vi "GetNodeHeirarchyArray_recursively.vi"(8 "error in (no error)":errorcluster, 9 "2D Array_All Paths":refnum<vi>, 10 "Nodes heirarchy IN (Leave EMPTY - used for recursion)":string[](array[string]), 11 "Node IN":refnum<k20>) -> (0 "error out":errorcluster)   [LabVIEW 2012]
doc: "SciScan 1.2 160622"
uses:
  <resource>/objmgr/DOMUserDefRef.rc
  <vilib>/xml/NI_XML.lvlib
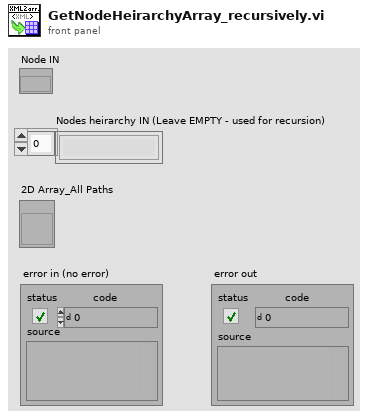
[diagram p1: front panel]
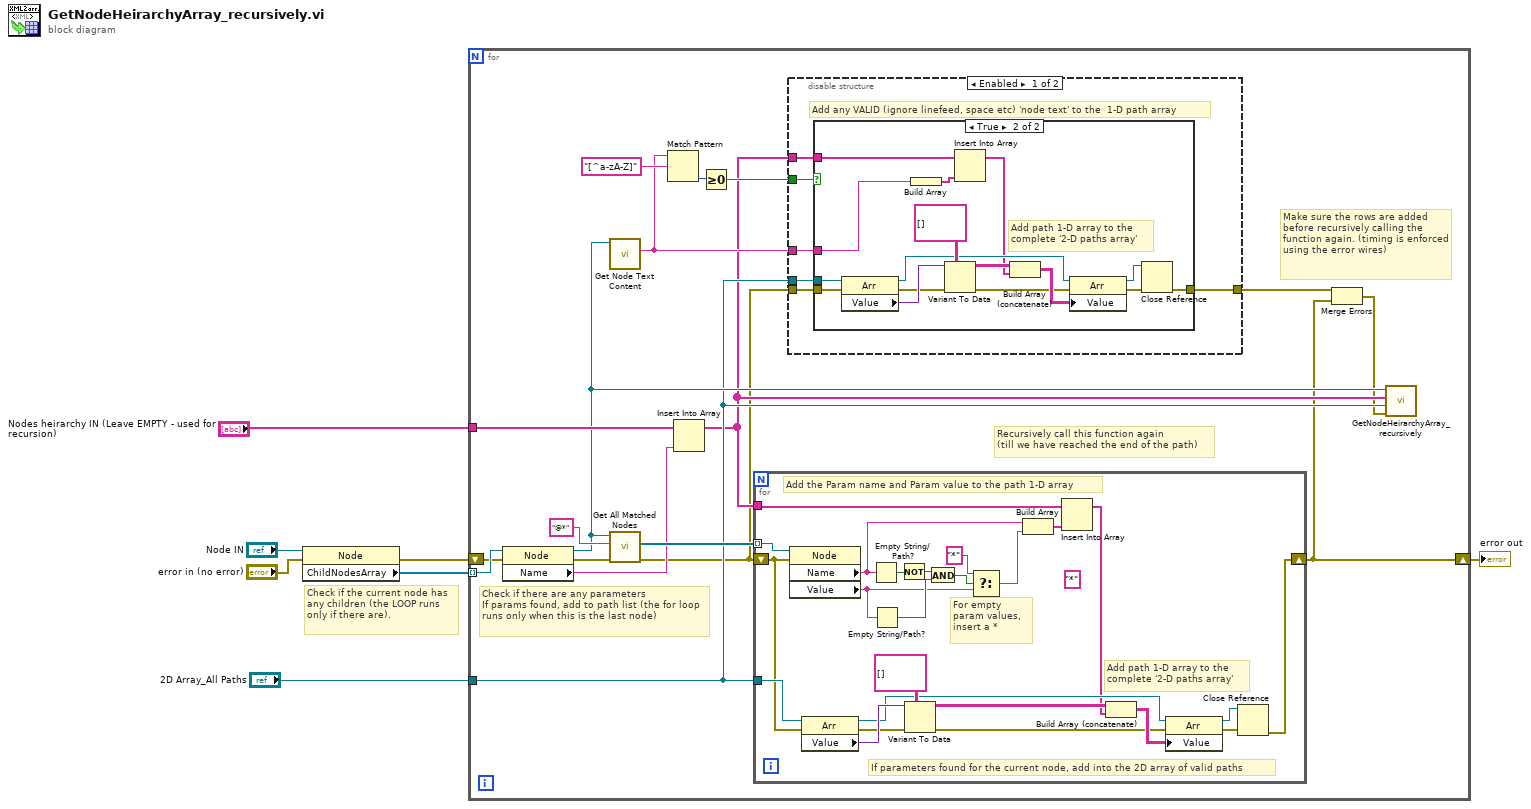
[diagram p0: block diagram]
diagram:
  # "Check if the current node has any children (the LOOP runs only if there are)."
  n1 = property class="Node"(reference="Node IN", error in="error in (no error)") -> (error out=w3:errorcluster, "ChildNodesArray"=w6:refnum<k20>[])  [unwired: 1 out]
  n2 = for {
    tunnel: w6 -> [w25] mode=indexing
    tunnel: "Nodes heirarchy IN (Leave EMPTY - used for recursion)" -> [w22]
    tunnel: "2D Array_All Paths" -> [w13]
    shift-right: [w9] -> w2
    shift-left: w3 -> [w21]
    # "Make sure the rows are added\nbefore recursively calling the function again. (timing is enforced using the error wires)"
    # "Recursively call this function again \n(till we have reached the end of the path)"
    # "Check if there are any parameters\nIf params found, add to path list (the for loop runs only when this is the last node)"
    n3 = property class="Node"(reference=w25, error in=w21) -> (reference out=w19:refnum<k20>, error out=w20:errorcluster, "Name"=w18:string)
    n4 = call <vilib>:"Get Node Text Content.vi"("node in"=w19) -> ("node text"=w16:string)  [unwired: 8 in, 2 out]
    n5 = call <vilib>:"Get All Matched Nodes.vi"("error in (no error)"=w20, "XPath expression"="@*", "node in"=w19) -> ("error out"=w11:errorcluster, "node result array"=w23:refnum<k20>[])  [unwired: 6 in, 1 out]
    n6 = Match Pattern(string=w16, regular expression="[^a-zA-Z]") -> (offset past match=w15:i32)  [unwired: 1 in, 3 out]
    n7 = Insert Into Array(array=w22, new element=w18) -> (w12:string[])  [unwired: 1 in]
    n8 = Greater Or Equal To 0?(x=w15) -> (x >= 0?=w14:bool)
    n9 = for {
      tunnel: w23 -> [w72] mode=indexing
      tunnel: w12 -> [w64]
      tunnel: w13 -> [w71]
      shift-right: [w58] -> w9
      shift-left: w11 -> [w61]
      (unwired) "*" ("t")
      # "For empty param values, insert a *"
      # "Add path 1-D array to the complete '2-D paths array'"
      # "Add the Param name and Param value to the path 1-D array"
      # "If parameters found for the current node, add into the 2D array of valid paths"
      n10 = property class="Node"(reference=w72, error in=w61) -> ("Name"=w56:string, "Value"=w51:string)  [unwired: 2 out]
      n11 = property class="Arr"(reference=w71, error in=w61) -> (reference out=w68:refnum<vi>, error out=w60:errorcluster, "Value"=w70:variant)
      n12 = Empty String/Path?(string/path=w56) -> (empty?=w55:bool)
      n13 = Empty String/Path?(string/path=w51) -> (empty?=w53:bool)
      n14 = Not(x=w55) -> (.not. x?=w54:bool)
      n15 = Variant To Data(error in=w60, type=string[][] [] ("Current Path Array"), Variant=w70) -> (data=w65:string[][], error out=w59:errorcluster)
      n16 = And(x=w54, y=w53) -> (x .and. y?=w52:bool)
      n17 = Select(t="*", s=w52, f=w51) -> (s? t:f=w49:string)
      n18 = Build Array(w56, w49) -> (w57:string[])
      n19 = Insert Into Array(array=w64, new element=w57) -> (w63:string[])  [unwired: 1 in]
      n20 = Build Array (concatenate)(w65, w63) -> (w62:string[][])
      n21 = property class="Arr"(reference=w68, error in=w59, "Value"=w62) -> (reference out=w66:refnum<vi>, error out=w67:errorcluster)
      n22 = Close Reference(reference=w66, error in (no error)=w67) -> (error out=w58:errorcluster)
    }
    n23 = disable-structure shown="Enabled" {
      disable-tunnel: w16 -> [w31 _]
      disable-tunnel: w14 -> [w30 _]
      disable-tunnel: w13 -> [w29 _]
      disable-tunnel: w12 -> [w28 _]
      disable-tunnel: w11 -> [w27 _]
      disable-tunnel: [w26 _] -> w10
      frame Enabled {
        # "Add any VALID (ignore linefeed, space etc) 'node text' to the  1-D path array"
        n24 = case shown="True" w30 {
          tunnel: w31 -> [_ w37]
          tunnel: w29 -> [_ w36]
          tunnel: w28 -> [_ w35]
          tunnel: w27 -> [w32 w34]
          tunnel: [w32 w33] -> w26
          frame False {
          }
          frame True {
            # "Add path 1-D array to the complete '2-D paths array'"
            n25 = property class="Arr"(reference=w36, error in=w34) -> (reference out=w46:refnum<vi>, error out=w39:errorcluster, "Value"=w48:variant)
            n26 = Build Array(w37) -> (w42:string[])
            n27 = Variant To Data(error in=w39, type=string[][] [] ("Current Path Array"), Variant=w48) -> (data=w43:string[][], error out=w38:errorcluster)
            n28 = Insert Into Array(array=w35, new element=w42) -> (w41:string[])  [unwired: 1 in]
            n29 = Build Array (concatenate)(w43, w41) -> (w40:string[][])
            n30 = property class="Arr"(reference=w46, error in=w38, "Value"=w40) -> (reference out=w44:refnum<vi>, error out=w45:errorcluster)
            n31 = Close Reference(reference=w44, error in (no error)=w45) -> (error out=w33:errorcluster)
          }
        }
      }
      frame Disabled {
      }
    }
    n32 = Merge Errors(w10, w9) -> (w8:errorcluster)
    n33 = call "GetNodeHeirarchyArray_recursively.vi"("error in (no error)"=w8, "2D Array_All Paths"=w13, "Nodes heirarchy IN (Leave EMPTY - used for recursion)"=w12, "Node IN"=w19) -> ()  [unwired: 7 in, 1 out]
  }
  "error out" <- w2
